vi "Disasemble 4-array bin.vi"(11 "4-Array Bin-Amp":dbl[](array[numeric])) -> (0 "Next Amp":dbl, 1 "Prev amp":dbl, 2 "Max amp":dbl, 3 "Max bin":i32)   [LabVIEW 2014]
doc: "This subVI is used to disassemble the 4-array composed by bin position and amplitudes"
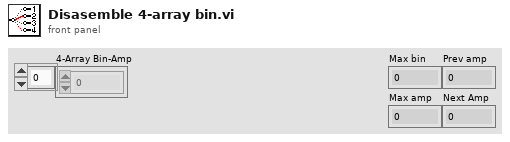
[diagram p1: front panel]
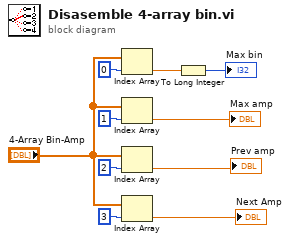
[diagram p0: block diagram]
diagram:
  n1 = Index Array(array="4-Array Bin-Amp", index=0) -> (element=w5:dbl)
  n2 = Index Array(array="4-Array Bin-Amp", index=1) -> (element=→"Max amp":dbl)
  n3 = Index Array(array="4-Array Bin-Amp", index=2) -> (element=→"Prev amp":dbl)
  n4 = Index Array(array="4-Array Bin-Amp", index=3) -> (element=→"Next Amp":dbl)
  n5 = To Long Integer(number=w5) -> (32bit integer=→"Max bin":i32)
